vi "DIM_DIO.ProcCases.vi"(0 "i ref in":refnum<vi>, 1 "selector":string, 2 "Data":T1, 3 "call cluster":T2={"Object"="", "Selector"="", "CallType"=enum."synchronous", "Async Object"="", "Async Selector"="", "Data Descriptor"="", "Data"=[], "Error #"=0, "Expire"=0}, 5 "error in (no error)":errorcluster) -> (14 "i ref out":refnum<vi>, 17 "answer cluster":T2={"Object"="", "Selector"="", "CallType"=enum."synchronous", "Async Object"="", "Async Selector"="", "Data Descriptor"="", "Data"=[], "Error #"=0, "Expire"=0}, 19 "error out":errorcluster)   [LabVIEW 2014, in "DIM_DIO.lvlib"]
doc: "This method is called by a process from within the default case in the event loop. The methods of a class that are linked to events will be called from THIS method. Add your code here."
uses:
  DIM_DIO.lvlib
  CS_Core/CSSystem/CoreDefs/CoreDefs.call_type.ctl
  CS_Core/BaseProcess/BaseProcess.descriptor string definition.ctl
  CS_Core/CSSystem/CoreDefs/CoreDefs.rawDataType.ctl
  CS_Core/CSSystem/CoreLib/CoreLib.string 2 byte array.vi
  CS_Core/CSSystem/CoreLib/CoreLib.byte array 2 short.vi
  CS_Core/CSSystem/CoreLib/CoreLib.byte array 2 int.vi
  CS_Core/CSSystem/CoreLib/CoreLib.lvlib
  CS_Core/BaseProcess/BaseProcess.lvlib
  CS_Core/CAEObj/CAEObj.lvlib
  CS_Core/CSApplicationBaseClasses/DigiIOBase/DigiIOBase.lvlib
  CS_Core/CSApplicationBaseClasses/DeviceBase/DeviceBase.lvlib
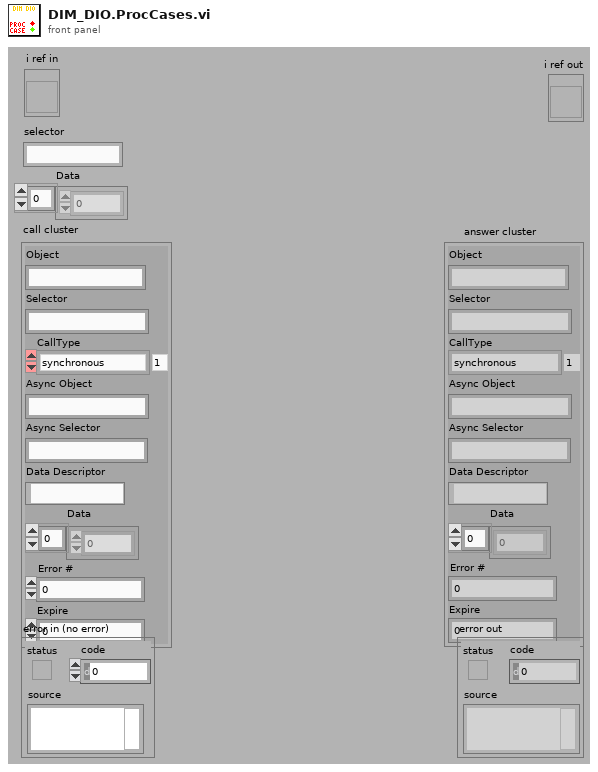
[diagram p1: front panel]
types:
  T1 = typedef "CoreDefs.rawDataType.ctl" = i8[]
  T2 = typedef "CoreDefs.call_type.ctl" = cluster{"Object":string, "Selector":string, "CallType":enum16{"simple", "synchronous", "asynchronous"}, "Async Object":string, "Async Selector":string, "Data Descriptor":T3, "Data":T1, "Error #":i32, "Expire":u32}
  T3 = typedef "BaseProcess.lvlib/BaseProcess.descriptor string definition.ctl" = string
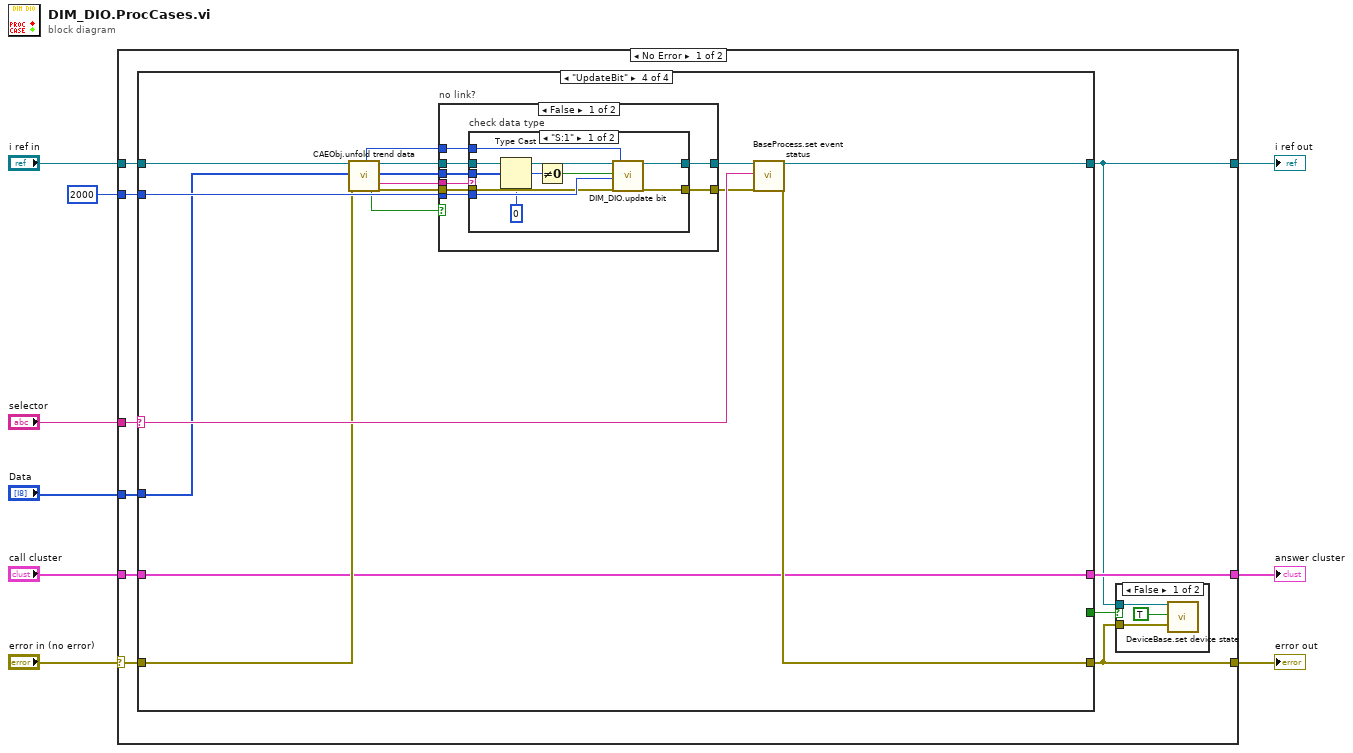
[diagram p0: block diagram]
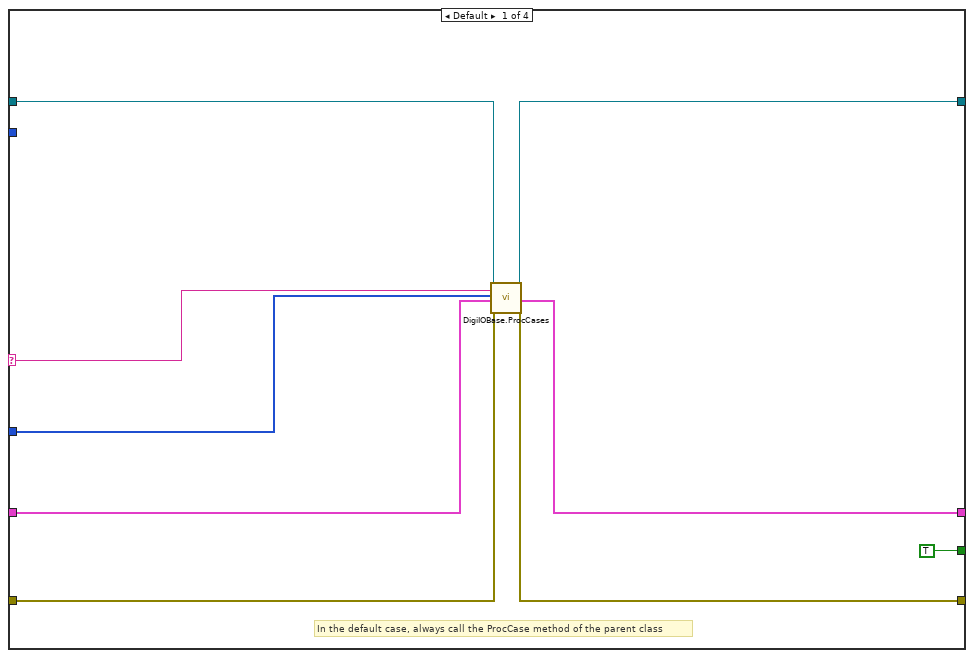
[diagram p3: hidden frame]
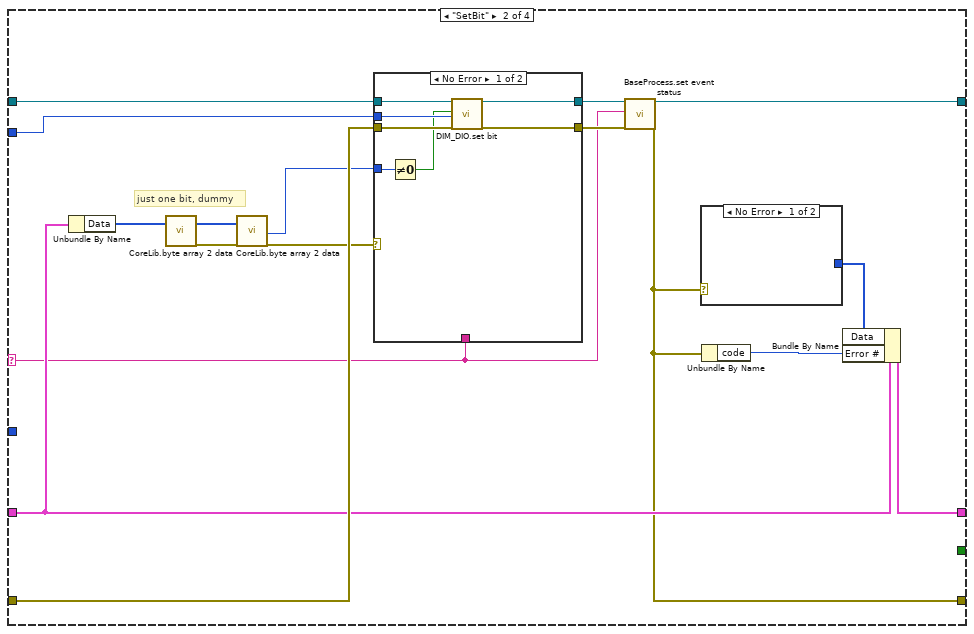
[diagram p4: hidden frame]
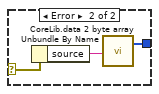
[diagram p5: hidden frame]
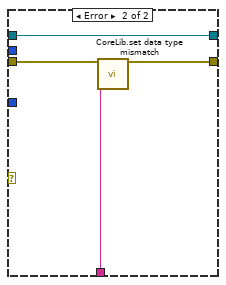
[diagram p6: hidden frame]
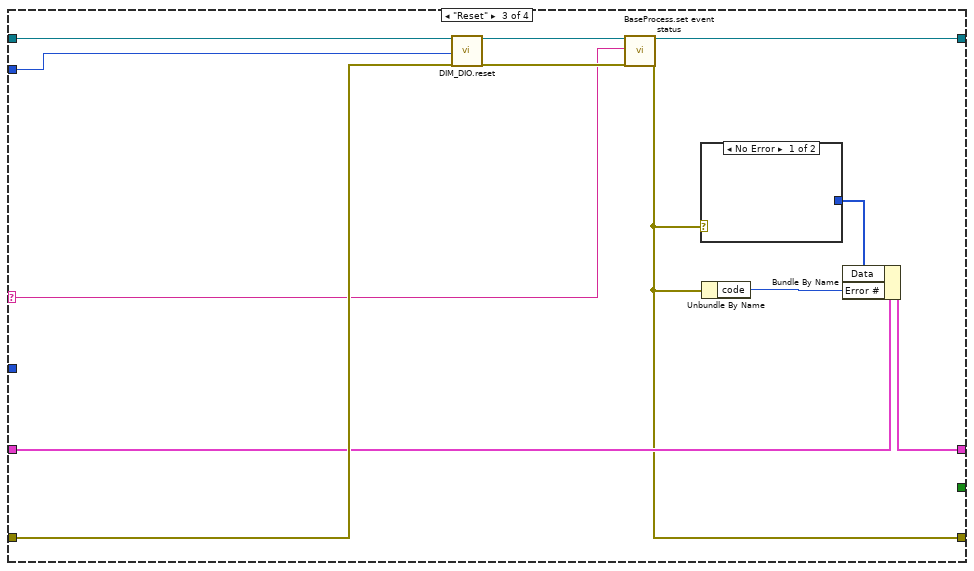
[diagram p7: hidden frame]
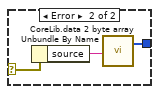
[diagram p8: hidden frame]
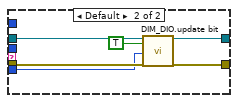
[diagram p9: hidden frame]
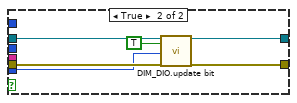
[diagram p10: hidden frame]
diagram:
  n1 = case shown="No Error" "error in (no error)" {
    selector: "error in (no error)" -> [w14 w124]
    tunnel: "selector" -> [w19 _]
    tunnel: [w18 w125] -> w8
    tunnel: "Data" -> [w17 _]
    tunnel: "call cluster" -> [w16 w125]
    tunnel: "i ref in" -> [w15 w126]
    tunnel: [w11 w126] -> w4
    tunnel: [w10 w124] -> w3
    tunnel: 2000 -> [w13 _]
    frame No Error {
      n2 = case shown="\"UpdateBit\"" w19 {
        selector: w19 -> [w25 w39 w65 w91]
        tunnel: w17 -> [w26 _ _ w79]
        tunnel: w15 -> [w24 w48 w74 w88]
        tunnel: [w31 w38 w64 w90] -> w11
        tunnel: w16 -> [w27 w45 w71 w78]
        tunnel: [w28 w44 w70 w78] -> w18
        tunnel: w14 -> [w30 w47 w73 w87]
        tunnel: [w29 w40 w66 w92] -> w10
        tunnel: w13 -> [_ w35 w63 w89]
        tunnel: [TRUE _ _ _] -> w12
        frame Default {
          # "In the default case, always call the ProcCase method of the parent class"
          n3 = call "DigiIOBase.ProcCases.vi"("i ref in"=w24, "selector"=w25, "Data"=w26, "call cluster"=w27, "error in (no error)"=w30) -> ("i ref out"=w31:refnum<vi>, "answer cluster"=w28:T2, "error out"=w29:errorcluster)  [unwired: 12 in]
        }
        frame "SetBit" {
          # "just one bit, dummy"
          n4 = Unbundle By Name(w45) -> ("Data"=w32:T1)
          n5 = call-poly "CoreLib.byte array 2 data.vi"("byteArray"=w32) -> ("byteArray out"=w34:T1, "error out"=w33:errorcluster)  [unwired: 16 in, 1 out]
          n6 = call-poly "CoreLib.byte array 2 data.vi"("byteArray"=w34, "error in (no error)"=w33) -> ("i16"=w37:i16, "error out"=w36:errorcluster)  [unwired: 15 in, 1 out]
          n7 = case shown="No Error" w36 {
            tunnel: [w57 w62] -> w42
            tunnel: w48 -> [w58 w62]
            tunnel: w47 -> [w55 w61]
            tunnel: [w54 w60] -> w41
            tunnel: w39 -> [_ w59]
            tunnel: w37 -> [w53 _]
            tunnel: w35 -> [w56 _]
            frame No Error {
              n8 = Not Equal To 0?(x=w53) -> (x != 0?=w52:bool)
              n9 = call "DIM_DIO.set bit.vi"("i ref in"=w58, "bitValue"=w52, "ms timeout (10000)"=w56, "error in (no error)"=w55) -> ("i ref out"=w57:refnum<vi>, "error out"=w54:errorcluster)  [unwired: 13 in, 1 out]
            }
            frame Error {
              n10 = call "CoreLib.set data type mismatch.vi"("error in (no error)"=w61, "error source"=w59) -> ("error out"=w60:errorcluster)  [unwired: 17 in]
            }
          }
          n11 = call "BaseProcess.set event status.vi"("i ref in"=w42, "EventStatus"=w39, "error in (no error)"=w41) -> ("i ref out"=w38:refnum<vi>, "error out"=w40:errorcluster)  [unwired: 14 in, 1 out]
          n12 = case shown="No Error" w40 {
            selector: w40 -> [_ w51]
            tunnel: [_ w50] -> w43
            frame No Error {
            }
            frame Error {
              n13 = Unbundle By Name(w51) -> ("source"=w49:string)
              n14 = call-poly "CoreLib.data 2 byte array.vi"("string"=w49) -> ("byteArray out"=w50:T1)  [unwired: 18 in]
            }
          }
          n15 = Unbundle By Name(w40) -> ("code"=w46:i32)
          n16 = Bundle By Name(cluster=w45, "Data"=w43, "Error #"=w46) -> (w44:T2)
        }
        frame "Reset" {
          n17 = call "DIM_DIO.reset.vi"("i ref in"=w74, "ms timeout (10000)"=w63, "error in (no error)"=w73) -> ("i ref out"=w68:refnum<vi>, "error out"=w67:errorcluster)  [unwired: 14 in, 1 out]
          n18 = call "BaseProcess.set event status.vi"("i ref in"=w68, "EventStatus"=w65, "error in (no error)"=w67) -> ("i ref out"=w64:refnum<vi>, "error out"=w66:errorcluster)  [unwired: 14 in, 1 out]
          n19 = case shown="No Error" w66 {
            selector: w66 -> [_ w77]
            tunnel: [_ w76] -> w69
            frame No Error {
            }
            frame Error {
              n20 = Unbundle By Name(w77) -> ("source"=w75:string)
              n21 = call-poly "CoreLib.data 2 byte array.vi"("string"=w75) -> ("byteArray out"=w76:T1)  [unwired: 18 in]
            }
          }
          n22 = Unbundle By Name(w66) -> ("code"=w72:i32)
          n23 = Bundle By Name(cluster=w71, "Data"=w69, "Error #"=w72) -> (w70:T2)
        }
        frame "UpdateBit" {
          n24 = call "CAEObj.unfold trend data.vi"("i ref in"=w88, "raw trend data"=w79, "error in (no error)"=w87) -> ("quality"=w80:i32, "no link"=w82:bool, "i ref out"=w85:refnum<vi>, "data"=w81:i8[], "typeDescriptor"=w86:string, "error out"=w84:errorcluster)  [unwired: 8 in, 3 out]
          n25 = case "no link?" shown="False" w82 {
            tunnel: [w101 w122] -> w93
            tunnel: w89 -> [w100 w118]
            tunnel: w86 -> [w99 _]
            tunnel: w85 -> [w98 w123]
            tunnel: w84 -> [w97 w121]
            tunnel: [w96 w120] -> w83
            tunnel: w81 -> [w95 _]
            tunnel: w80 -> [w94 _]
            frame False {
              n26 = case "check data type" shown="\"S:1\"" w99 {
                tunnel: [w110 w116] -> w101
                tunnel: w98 -> [w111 w117]
                tunnel: w97 -> [w108 w115]
                tunnel: w100 -> [w109 w112]
                tunnel: [w107 w114] -> w96
                tunnel: w95 -> [w106 _]
                tunnel: w94 -> [w102 _]
                frame "S:1" {
                  n27 = Type Cast(type=i16 0, x=w106) -> (*(type *) &x=w104:i16)
                  n28 = Not Equal To 0?(x=w104) -> (x != 0?=w103:bool)
                  n29 = call "DIM_DIO.update bit.vi"("i ref in"=w111, "bitValue"=w103, "ms timeout (10000)"=w109, "error in (no error)"=w108, "bitQuality"=w102) -> ("i ref out"=w110:refnum<vi>, "error out"=w107:errorcluster)  [unwired: 12 in, 1 out]
                }
                frame Default {
                  n30 = call "DIM_DIO.update bit.vi"("i ref in"=w117, "badValue"=TRUE, "ms timeout (10000)"=w112, "error in (no error)"=w115) -> ("i ref out"=w116:refnum<vi>, "error out"=w114:errorcluster)  [unwired: 13 in, 1 out]
                }
              }
            }
            frame True {
              n31 = call "DIM_DIO.update bit.vi"("i ref in"=w123, "badValue"=TRUE, "ms timeout (10000)"=w118, "error in (no error)"=w121) -> ("i ref out"=w122:refnum<vi>, "error out"=w120:errorcluster)  [unwired: 13 in, 1 out]
            }
          }
          n32 = call "BaseProcess.set event status.vi"("i ref in"=w93, "EventStatus"=w91, "error in (no error)"=w83) -> ("i ref out"=w90:refnum<vi>, "error out"=w92:errorcluster)  [unwired: 14 in, 1 out]
        }
      }
      n33 = case shown="False" w12 {
        tunnel: w11 -> [w21 _]
        tunnel: w10 -> [w20 _]
        frame False {
          n34 = call "DeviceBase.set device state.vi"("i ref in"=w21, "implicit"=TRUE, "device error"=w20) -> ()  [unwired: 14 in, 3 out]
        }
        frame True {
        }
      }
    }
    frame Error {
    }
  }
  "answer cluster" <- w8
  "i ref out" <- w4
  "error out" <- w3
